vi "Wait for Ready.vi"(0 "Notifier Name":string, 11 "Error In":errorcluster) -> (4 "Notifier Name Out":string, 8 "Ready?":bool, 15 "Error Out":errorcluster)   [LabVIEW 2020]
uses:
  Hardware Configuration/Hardware Configuration Controls/Company.ctl
  Photometrics/Prime BSI/PVCam LabView/Prime BSI Type Defs/Prime BSI Notifier Element.ctl
  Photometrics/Prime BSI/PVCam LabView/Prime BSI Type Defs/Prime BSI Actions.ctl
  Photometrics/Prime BSI/PVCam LabView/Prime BSI Type Defs/Prime BSI Parameters.ctl
  Photometrics/Prime BSI/PVCam LabView/Prime BSI Type Defs/Prime BSI Parameter List.ctl
  Photometrics/Prime BSI/PVCam LabView/Prime BSI Type Defs/Prime BSI ROI.ctl
  <vilib>/vision/Image Controls.llb/IMAQ Image.ctl
  Hamamatsu/Orca Flash/Orca Flash Controls/Orca Flash Notifier Element.ctl
  Hamamatsu/Orca Flash/Orca Flash Controls/Orca Flash Actions.ctl
  Hamamatsu/Orca Flash/Orca Flash Controls/Orca Flash Parameters.ctl
  Hamamatsu/Orca Flash/Orca Flash Controls/Orca Flash Parameter List.ctl
  Hamamatsu/Orca Flash/Orca Flash Controls/Orca Flash ROI.ctl
  IDS/IDS Controls/IDS Notifier Element.ctl
  IDS/IDS Controls/IDS Actions.ctl
  IDS/IDS Controls/IDS Parameters.ctl
  IDS/IDS Controls/IDS Parameter List.ctl
  IDS/IDS Controls/IDS ROI.ctl
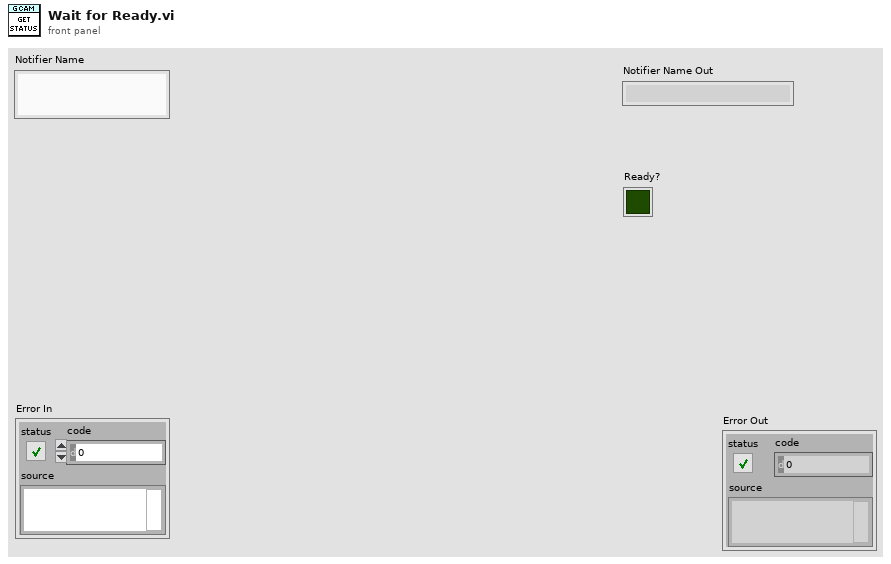
[diagram p1: front panel]
types:
  T1 = typedef "Company.ctl" = enum16{"AA Opto Electronic", "ASI", "Coherent", "Creset Optics", "CVI", "DAQmx", "Hamamatsu", "IDS", "Mad City Labs", "Marzhauser", "Measurement Computing", "MPB Com", "Photometrics", "PI", "Prior", "Thorlabs"}
  T2 = typedef "Prime BSI Notifier Element.ctl" = cluster{"PVCam Actions":T3, "Received?":bool, "PVCam Parameter":T4, "PVCam ROI":T6, "Running?":bool, "File Path":path, "# of frames":u32, "Image Ref":T7, "Binning":i32}
  T3 = typedef "Prime BSI Actions.ctl" = enum16{"Do Nothing", "Preview", "Record", "Abort", "Record Settings", "Set Parameter", "Get Parameter", "Set ROI", "Get ROI", "Status", "Quit"}
  T4 = typedef "Prime BSI Parameters.ctl" = cluster{"Parameter":T5, "Value":string[]}
  T5 = typedef "Prime BSI Parameter List.ctl" = enum16{"Exposure Time (s)", "Binning", "Readout Port List", "Available Gain List"}
  T6 = typedef "Prime BSI ROI.ctl" = cluster{"H Offset":i32, "V Offset":i32, "H Width":i32, "V Width":i32}
  T7 = typedef "IMAQ Image.ctl" = refnum<image>
  T8 = typedef "Orca Flash Notifier Element.ctl" = cluster{"Camera Actions":T9, "Received?":bool, "Running?":bool, "sCMOS Parameter":T10, "sCMOS ROI":T12, "Save Path":path, "# of frames":u32, "Image Ref":T7}
  T9 = typedef "Orca Flash Actions.ctl" = enum16{"IDLE", "PREVIEW", "RECORD", "Record Settings", "SETPARAM", "GETPARAM", "SETROI", "GETROI", "PROGRESSIVE MODE", "AREA MODE", "STATUS", "QUIT"}
  T10 = typedef "Orca Flash Parameters.ctl" = cluster{"Value":dbl, "Parameter":T11}
  T11 = typedef "Orca Flash Parameter List.ctl" = u32
  T12 = typedef "Orca Flash ROI.ctl" = cluster{"H Offset":i32, "V Offset":i32, "H Width":i32, "V Width":i32}
  T13 = typedef "IDS Notifier Element.ctl" = cluster{"IDS Actions":T14, "Received?":bool, "IDS Parameter":T15, "IDS ROI":T17, "Running?":bool, "File Path":path, "# of frames":u32, "Image Ref":T7, "Error":errorcluster, "Binning":i32}
  T14 = typedef "IDS Actions.ctl" = enum16{"Error Check", "Initialize", "Preview", "Record", "Abort", "Record Settings", "Set Parameter", "Get Parameter", "Set ROI", "Get ROI", "Status", "Quit"}
  T15 = typedef "IDS Parameters.ctl" = cluster{"Parameter":T16, "Value":dbl}
  T16 = typedef "IDS Parameter List.ctl" = enum16{"Exposure Time (s)", "Binning"}
  T17 = typedef "IDS ROI.ctl" = cluster{"H Offset":i32, "V Offset":i32, "H Width":i32, "V Width":i32}
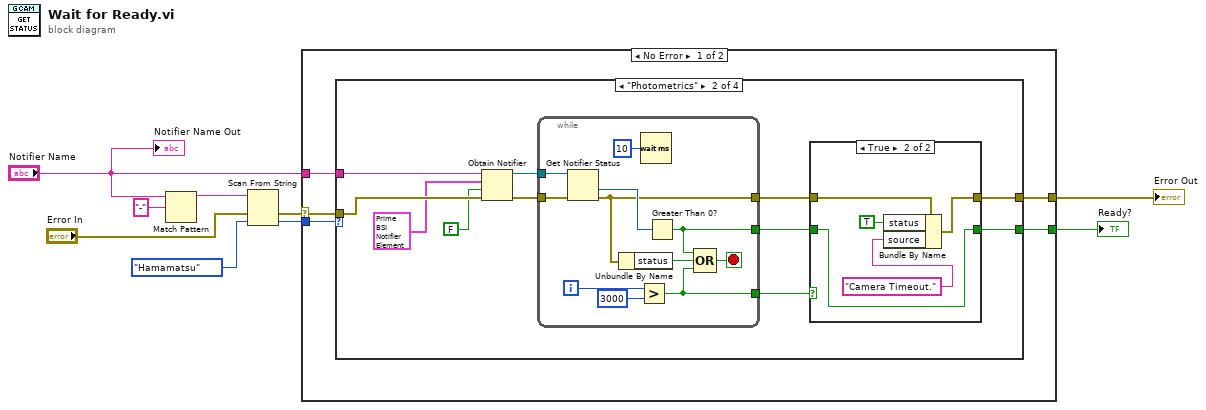
[diagram p0: block diagram]
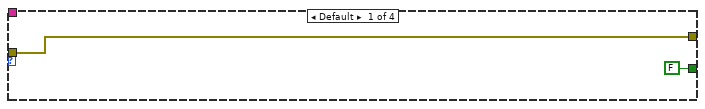
[diagram p2: hidden frame]
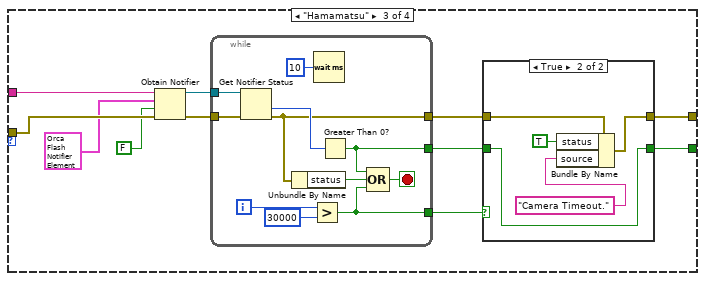
[diagram p4: hidden frame]
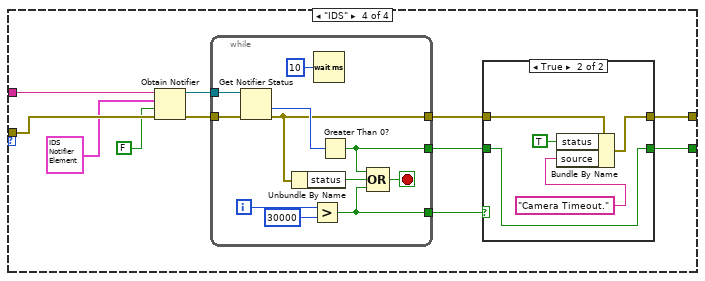
[diagram p6: hidden frame]
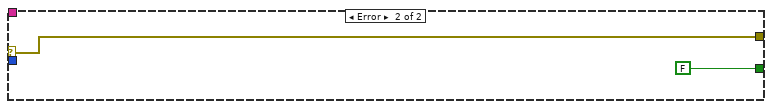
[diagram p8: hidden frame]
diagram:
  n1 = Match Pattern(string="Notifier Name", regular expression="-") -> (before substring=w7:string)  [unwired: 1 in, 3 out]
  n2 = Scan From String(input string=w7, error in="Error In", default 1=Company."Hamamatsu" ("Company")) -> (error out=w4:errorcluster, output 1=w6:T1)  [unwired: 2 in, 2 out]
  n3 = case shown="No Error" w4 {
    selector: w4 -> [w12 w105]
    tunnel: w6 -> [w14 _]
    tunnel: "Notifier Name" -> [w13 _]
    tunnel: [w11 FALSE] -> w2
    tunnel: [w10 w105] -> w1
    frame No Error {
      n4 = case shown="\"Photometrics\"" w14 {
        tunnel: w13 -> [_ w27 w56 w85]
        tunnel: w12 -> [w16 w26 w55 w84]
        tunnel: [FALSE w19 w48 w77] -> w11
        tunnel: [w16 w17 w46 w75] -> w10
        frame Default {
        }
        frame "Photometrics" {
          n5 = Obtain Notifier(name (unnamed)=w27, notification data type=T2 {"PVCam Actions"=enum."Do Nothing", "Received?"=FALSE, "PVCam Parameter"={"Parameter"=enum."Exposure Time (s)", "Value"=[]}, "PVCam ROI"={"H Offset"=0, "V Offset"=0, "H Width"=0, "V Width"=0}, "Running?"=FALSE, "File Path"=path "", "# of frames"=0, "Image Ref"=refnum, "Binning"=0} ("PVCam Camera Cluster"), create if not found? (T)=FALSE, error in (no error)=w26) -> (notifier out=w23:refnum<notifier>, error out=w22:errorcluster)  [unwired: 1 out]
          n6 = while {
            tunnel: w23 -> [w45]
            tunnel: w22 -> [w44]
            tunnel: [w42] -> w18
            tunnel: [w36] -> w20
            tunnel: [w35] -> w21
            i -> [w40]
            stop <- w37 stop-if-true
            n7 = Get Notifier Status(notifier=w45, error in (no error)=w44) -> (# waiting=w43:i32, error out=w42:errorcluster)  [unwired: 3 out]
            n8 = Unbundle By Name(w42) -> ("status"=w38:bool)
            n9 = Greater?(x=w40, y=3000) -> (0:w35:bool)
            n10 = Wait (ms)(milliseconds to wait=u32 10) -> ()  [unwired: 1 out]
            n11 = Greater Than 0?(x=w43) -> (x > 0?=w36:bool)
            n12 = Compound Arithmetic op=OR(w36, w38, w35) -> (w37:bool)
          }
          n13 = case shown="True" w21 {
            tunnel: w20 -> [w29 w34]
            tunnel: [w29 w34] -> w19
            tunnel: w18 -> [w28 w33]
            tunnel: [w28 w31] -> w17
            frame False {
            }
            frame True {
              n14 = Bundle By Name(cluster=w33, "status"=TRUE, "source"="Camera Timeout.") -> (w31:errorcluster)
            }
          }
        }
        frame "Hamamatsu" {
          n15 = Obtain Notifier(name (unnamed)=w56, notification data type=T8 {"Camera Actions"=enum."IDLE", "Received?"=FALSE, "Running?"=FALSE, "sCMOS Parameter"={"Value"=0.0, "Parameter"=0}, "sCMOS ROI"={"H Offset"=0, "V Offset"=0, "H Width"=0, "V Width"=0}, "Save Path"=path "", "# of frames"=0, "Image Ref"=refnum} ("Camera Cluster"), create if not found? (T)=FALSE, error in (no error)=w55) -> (notifier out=w52:refnum<notifier>, error out=w51:errorcluster)  [unwired: 1 out]
          n16 = while {
            tunnel: w52 -> [w74]
            tunnel: w51 -> [w73]
            tunnel: [w71] -> w47
            tunnel: [w65] -> w49
            tunnel: [w64] -> w50
            i -> [w69]
            stop <- w66 stop-if-true
            n17 = Get Notifier Status(notifier=w74, error in (no error)=w73) -> (# waiting=w72:i32, error out=w71:errorcluster)  [unwired: 3 out]
            n18 = Unbundle By Name(w71) -> ("status"=w67:bool)
            n19 = Greater?(x=w69, y=30000) -> (0:w64:bool)
            n20 = Wait (ms)(milliseconds to wait=u32 10) -> ()  [unwired: 1 out]
            n21 = Greater Than 0?(x=w72) -> (x > 0?=w65:bool)
            n22 = Compound Arithmetic op=OR(w65, w67, w64) -> (w66:bool)
          }
          n23 = case shown="True" w50 {
            tunnel: w49 -> [w58 w63]
            tunnel: [w58 w63] -> w48
            tunnel: w47 -> [w57 w62]
            tunnel: [w57 w60] -> w46
            frame False {
            }
            frame True {
              n24 = Bundle By Name(cluster=w62, "status"=TRUE, "source"="Camera Timeout.") -> (w60:errorcluster)
            }
          }
        }
        frame "IDS" {
          n25 = Obtain Notifier(name (unnamed)=w85, notification data type=T13 {"IDS Actions"=enum."Error Check", "Received?"=FALSE, "IDS Parameter"={"Parameter"=enum."Exposure Time (s)", "Value"=0.0}, "IDS ROI"={"H Offset"=0, "V Offset"=0, "H Width"=0, "V Width"=0}, "Running?"=FALSE, "File Path"=path "", "# of frames"=0, "Image Ref"=refnum, "Error"={"status"=FALSE, "code"=0, "source"=""}, "Binning"=0} ("IDS Camera Cluster"), create if not found? (T)=FALSE, error in (no error)=w84) -> (notifier out=w81:refnum<notifier>, error out=w80:errorcluster)  [unwired: 1 out]
          n26 = while {
            tunnel: w81 -> [w103]
            tunnel: w80 -> [w102]
            tunnel: [w100] -> w76
            tunnel: [w94] -> w78
            tunnel: [w93] -> w79
            i -> [w98]
            stop <- w95 stop-if-true
            n27 = Get Notifier Status(notifier=w103, error in (no error)=w102) -> (# waiting=w101:i32, error out=w100:errorcluster)  [unwired: 3 out]
            n28 = Unbundle By Name(w100) -> ("status"=w96:bool)
            n29 = Greater?(x=w98, y=30000) -> (0:w93:bool)
            n30 = Wait (ms)(milliseconds to wait=u32 10) -> ()  [unwired: 1 out]
            n31 = Greater Than 0?(x=w101) -> (x > 0?=w94:bool)
            n32 = Compound Arithmetic op=OR(w94, w96, w93) -> (w95:bool)
          }
          n33 = case shown="True" w79 {
            tunnel: w78 -> [w87 w92]
            tunnel: [w87 w92] -> w77
            tunnel: w76 -> [w86 w91]
            tunnel: [w86 w89] -> w75
            frame False {
            }
            frame True {
              n34 = Bundle By Name(cluster=w91, "status"=TRUE, "source"="Camera Timeout.") -> (w89:errorcluster)
            }
          }
        }
      }
    }
    frame Error {
    }
  }
  "Error Out" <- w1
  "Ready?" <- w2
  "Notifier Name Out" <- "Notifier Name"
